vi "testEXT Passes If Element Is Found At Given Index.vi"(8 "error in (no error)":errorcluster, 11 "TestCase in":refnum<class "Search In 1D Array Test Case.lvclass">) -> (0 "error out":errorcluster, 3 "TestCase out":refnum<class "Search In 1D Array Test Case.lvclass">)   [LabVIEW 2015, in "Search In 1D Array Test Case.lvclass"]
uses:
  Search In 1D Array Test Case.lvclass
  SubVIs/Search in array/Pass If In 1D Array (EXT).vi
  <vilib>/addons/_JKI Toolkits/VI Tester/TestCase.llb/TestCase.lvclass
  VITAC.lvlib
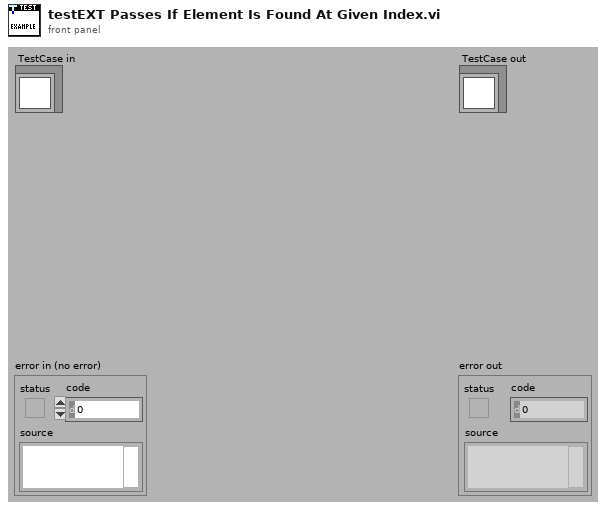
[diagram p1: front panel]
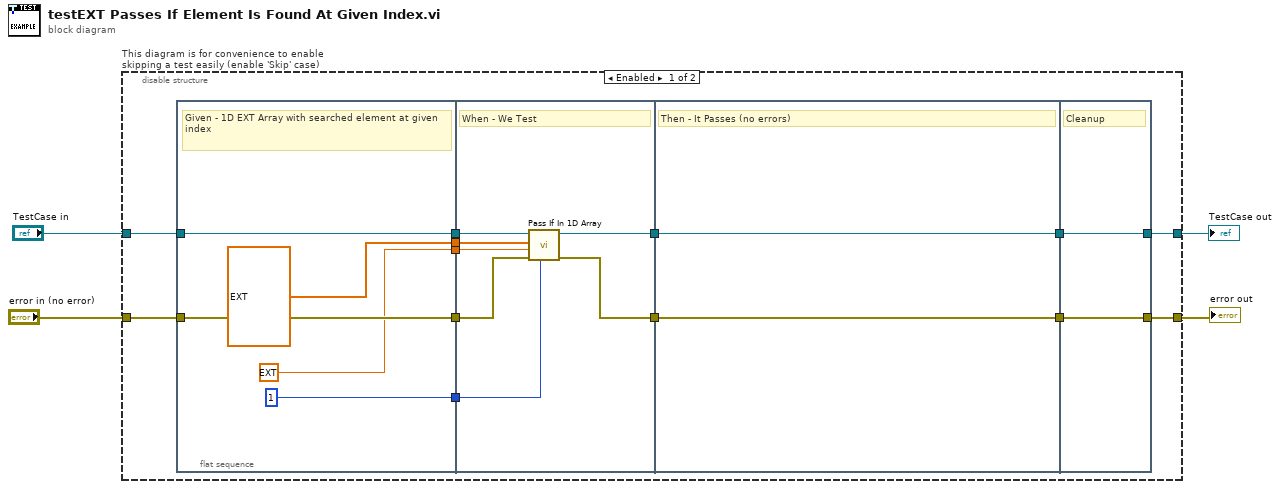
[diagram p0: block diagram]
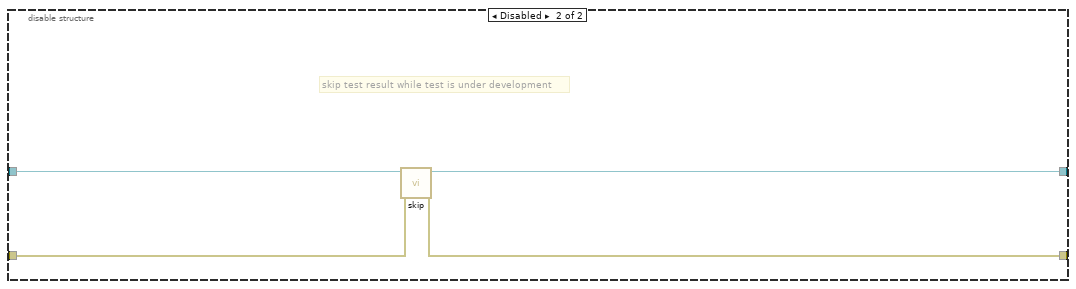
[diagram p2: hidden frame]
diagram:
  n1 = disable-structure "This diagram is for convenience to enable skipping a test easily (enable 'Skip' case)" shown="Enabled" {
    disable-tunnel: "TestCase in" -> [w9 w37]
    disable-tunnel: [w12 w35] -> w1
    disable-tunnel: [w11 w36] -> w3
    disable-tunnel: "error in (no error)" -> [w10 w34]
    frame Enabled {
      n2 = flat-sequence {
        tunnel: w10 -> [w21]
        tunnel: w9 -> [w22]
        tunnel: [w22] -> w17
        tunnel: [w21] -> w16
        tunnel: [ext 5.0] -> w7
        tunnel: [ext[] [1.0, 5.0, 10.0, 20.5]] -> w6
        tunnel: [1] -> w5
        tunnel: [w28] -> w15
        tunnel: [w27] -> w14
        tunnel: w17 -> [w29]
        tunnel: w16 -> [w26]
        tunnel: w7 -> [w25]
        tunnel: w6 -> [w24]
        tunnel: w5 -> [w23]
        tunnel: [w31] -> w13
        tunnel: w15 -> [w31]
        tunnel: w14 -> [w30]
        tunnel: [w30] -> w8
        tunnel: [w32] -> w11
        tunnel: [w33] -> w12
        tunnel: w13 -> [w33]
        tunnel: w8 -> [w32]
        frame #0 {
          # "Given - 1D EXT Array with searched element at given index"
        }
        frame #1 {
          # "When - We Test"
          n3 = call-poly "Pass If In 1D Array.vi"("expected index (optional)"=w23, "error in (no error)"=w26, "element"=w25, "1D array"=w24, "TestCase in"=w29) -> ("error out"=w27:errorcluster, "TestCase out"=w28:refnum<class "Search In 1D Array Test Case.lvclass">)  [unwired: 5 in]
        }
        frame #2 {
          # "Then - It Passes (no errors)"
        }
        frame #3 {
          # "Cleanup"
        }
      }
    }
    frame Disabled {
      # "skip test result while test is under development"
      n4 = call <vilib>:"skip.vi"("error in (no error)"=w34, "TestCase in"=w37) -> ("error out"=w36:errorcluster, "TestCase out"=w35:refnum<class "Search In 1D Array Test Case.lvclass">)  [unwired: 8 in]
    }
  }
  "error out" <- w3
  "TestCase out" <- w1
